vi "Create All Message Queues.vi"(8 "error in (no error)":T1 caption="entrée d'erreur (pas d'erreur)", 11 "Événement utilisateur - Arrêt":refnum<user-event>) -> (0 "error out":T1 caption="sortie d'erreur", 3 "Files d'attente de messages en sortie":T2)   [LabVIEW 2020, in "Message Queue.lvlib"]
doc: "Ce VI crée et initialise toutes les files d'attente de messages de l'application. Si votre application requiert plusieurs files d'attente de messages, cliquez sur la constante \"Message Queues\" ci-dessus avec le bouton droit et sélectionnez Ouvrir la déf. de type. Ajoutez les nouvelles files d'attente de messages à la définition de type puis initialisez-les dans ce VI."
uses:
  Message Queue.lvlib
  All Message Queues.ctl
  Message Cluster.ctl
  Enqueue Message (Single).vi
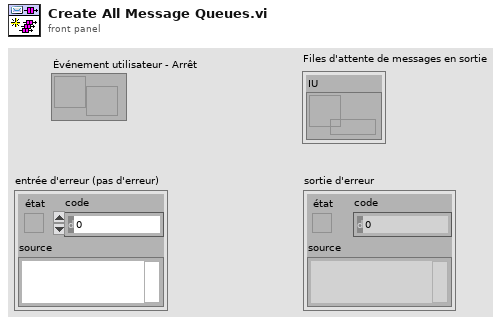
[diagram p1: front panel]
types:
  T1 = cluster{"état":bool, "code":i32, "source":string}
  T2 = typedef "Message Queue.lvlib/All Message Queues.ctl" = cluster{"IU":refnum<queue>}
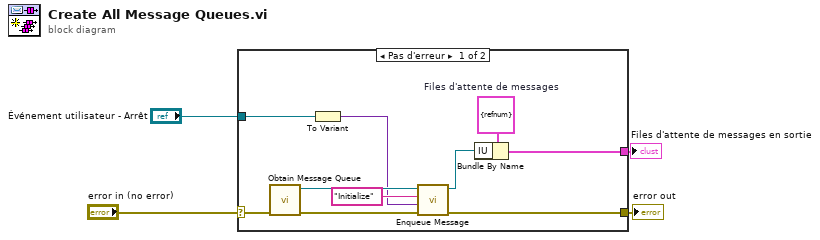
[diagram p0: block diagram]
diagram:
  n1 = case shown="Pas d'erreur" "error in (no error)" {
    selector: "error in (no error)" -> [w11 w15]
    tunnel: [w14 w15] -> w4
    tunnel: [w12 _] -> w3
    tunnel: "Événement utilisateur - Arrêt" -> [w6 _]
    frame No Error {
      w13 = T2 {"IU"=refnum}  # Files d'attente de messages
      n2 = call "Obtain Message Queue.vi"("error in (no error)"=w11) -> ("error out"=w10:T1, "File d'attente de messages"=w8:refnum<queue>)  [unwired: 9 in]
      n3 = To Variant(anything=w6) -> (Variant=w5:variant)
      n4 = call-poly "Enqueue Message.vi"("error in (no error)"=w10, "Données de message"=w5, "Message"="Initialize", "File d'attente de messages"=w8) -> ("error out"=w14:T1, "File d'attente de message dup."=w7:refnum<queue>)  [unwired: 6 in]
      n5 = Bundle By Name(cluster=w13, "IU"=w7) -> (w12:T2)
    }
    frame Error {
    }
  }
  "Files d'attente de messages en sortie" <- w3
  "error out" <- w4
